vi "Polling Core.vi"(8 "Error In":errorcluster, 11 "BNT_DAQmx-MCSV-DOPWM in":refnum<class "BNT_DAQmx-MCSV-DOPWM.lvclass">) -> (0 "Error Out":errorcluster, 3 "BNT_DAQmx-MCSV-DOPWM out":refnum<class "BNT_DAQmx-MCSV-DOPWM.lvclass">)   [LabVIEW 2017, in "BNT_DAQmx.lvlib" / "BNT_DAQmx-MCSV-DOPWM.lvclass"]
uses:
  BNT_DAQmx-MCSV-DOPWM.lvclass
  C:/User/Brand/LVP/Acc/VacuumHeating/Packages/BNT_DAQmx/BNT_DAQmx-MCSV/BNT_DAQmx-MCSV.lvclass
  BNT_DAQmx-MCSV-DOPWM.lvclass/BNT_DAQmx-MCSV-DOPWM.ctl
  <vilib>/Waveform/WDTOps.llb/WDT Get Waveform Subset DBL.vi
  <vilib>/Waveform/WDTOps.llb/WDT Get XY Value DBL.vi
  BNT_DAQmx-MCSV/BNT_DAQmx-MCSV.lvclass
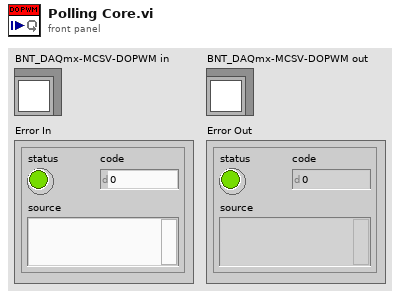
[diagram p1: front panel]
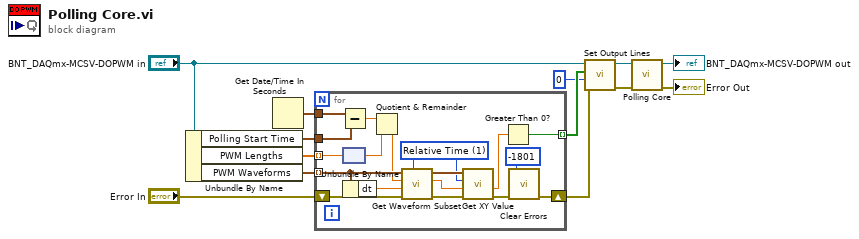
[diagram p0: block diagram]
diagram:
  n1 = Unbundle By Name("BNT_DAQmx-MCSV-DOPWM in") -> ("Polling Start Time"=w1:timestamp, "PWM Lengths"=w3:dbl[unit][], "PWM Waveforms"=w4:waveform(dbl)[])
  n2 = Get Date/Time In Seconds() -> (seconds since 1Jan1904=w5:timestamp)
  n3 = for {
    tunnel: w4 -> [w31] mode=indexing
    shift-right: [w18] -> w8
    shift-left: "Error In" -> [w28]
    tunnel: [w21] -> w7 mode=indexing
    tunnel: w5 -> [w16]
    tunnel: w3 -> [w15] mode=indexing
    tunnel: w1 -> [w14]
    w23 = u16 1 items=["Samples", "Relative Time"] ("start/duration format")
    n4 = Subtract(x=w16, y=w14) -> (x-y=w30:dbl)
    n5 = node(w15) -> (w19:dbl)
    n6 = Unbundle By Name(w31) -> ("dt"=w29:dbl)
    n7 = Quotient & Remainder(x=w30, y=w19) -> (x-y*floor(x/y)=w20:dbl)  [unwired: 1 out]
    n8 = call-poly <vilib>:"Get Waveform Subset.vi"("start/duration format"=w23, "error in (no error)"=w28, "duration"=w29, "start samples/time"=w20, "waveform in"=w31) -> ("error out"=w26:errorcluster, "actual start samples/time"=w24:dbl, "waveform out"=w27:waveform(dbl))  [unwired: 1 in, 1 out]
    n9 = call-poly <vilib>:"Get XY Value.vi"("error in (no error)"=w26, "Y position"=w24, "Y position format"=w23, "waveform in"=w27) -> ("error out"=w25:errorcluster, "Y value"=w22:dbl)  [unwired: 3 in, 3 out]
    n10 = Greater Than 0?(x=w22) -> (x > 0?=w21:bool)
    n11 = call <vilib>:"Clear Errors.vi"("error in (no error)"=w25, "specific error code to clear (0: all)"=-1801) -> ("error out"=w18:errorcluster)  [unwired: 4 in, 1 out]
  }
  n12 = call "Set Output Lines.vi"("Error In"=w8, "Start Index"=0, "DO Lines"=w7, "BNT_DAQmx-MCSV in"="BNT_DAQmx-MCSV-DOPWM in") -> ("Error Out"=w10:errorcluster, "BNT_DAQmx-MCSV out"=w11:refnum<class "BNT_DAQmx-MCSV-DOPWM.lvclass">)  [unwired: 6 in]
  n13 = call-parent "Polling Core.vi"("Error In"=w10, "BNT_DAQmx-MCSV in"=w11) -> ("Error Out"=→"Error Out":errorcluster, "BNT_DAQmx-MCSV out"=→"BNT_DAQmx-MCSV-DOPWM out":refnum<class "BNT_DAQmx-MCSV-DOPWM.lvclass">)  [unwired: 8 in]
